vi "SAOMM-QueryHexapod.vi"(0 "PRAMMS-COMM IN":refnum<visa-resource-name>="Hp\u0000\u0002", 2 "Bool Refnum":refnum<vi>, 7 "Signature":u32=1886544237, 11 "Error IN":errorcluster, 13 "EnumMessageType":cluster{"Type":string[], "Enum":u32[]}={"Type"=["emtError", "emtAreYouThere", "emtAcknowledgment", "emtGetClientType", "emtClientType", "emtGetImageExposureTime", "emtSetImageExposureTime", "emtImageExposureTime", "emtGetOptimalExposureTime", "emtSetOptimalExposureTime", "emtOptimalExposureTime", "emtGetImageEMGain", "emtSetImageEMGain", "emtImageEMGain", "emtGetFPGACtrl", "emtSetFPGACtrl", "emtFPGACtrl", "emtGetImageWidth", "emtSetImageWidth", "emtImageWidth", "emtGetImageHeight", "emtSetImageHeight", "emtImageHeight", "emtGetImageBinning", "emtSetImageBinning", "emtImageBinning", "emtGetImageDisplayFrameRate", "emtSetImageDisplayFrameRate", "emtImageDisplayFrameRate", "emtGetROIWidth", "emtSetROIWidth", "emtROIWidth", "emtGetROIHeight", "emtSetROIHeight", "emtROIHeight", "emtGetROIXOffset", "emtSetROIXOffset", "emtROIXOffset", "emtGetROIYOffset", "emtSetROIYOffset", "emtROIYOffset", "emtStartAcquisition", "mtStopAcquisition", "emtAcquisitionStarted", "emtAcquisitionStopped", "emtGetFalconImage", "emtFalconImage"], "Enum"=[1, 2, 3, 4, 5, 1001, 1101, 1201, 1002, 1102, 1202, 1003, 1103, 1203, 1004, 1104, 1204, 1005, 1105, 1205, 1006, 1106, 1206, 1007, 1107, 1207, 1008, 1108, 1208, 1009, 1109, 1209, 1010, 1110, 1210, 1011, 1111, 1211, 1012, 1112, 1212, 1130, 1131, 1150, 1151, 1070, 1270]}) -> (4 "PRAMMS-COMM OUT":refnum<visa-resource-name>, 15 "Error OUT":errorcluster)   [LabVIEW 2019]
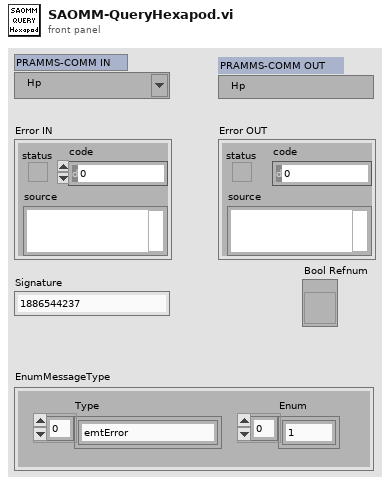
[diagram p1: front panel]
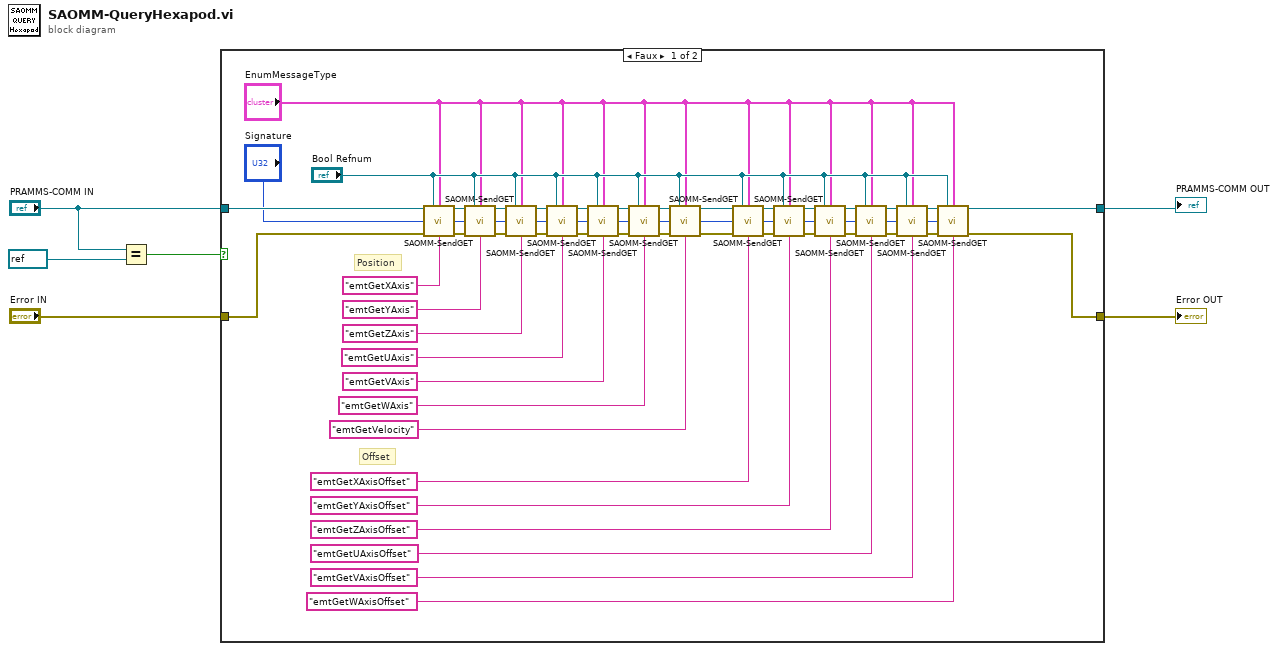
[diagram p0: block diagram]
diagram:
  n1 = Equal?(x="PRAMMS-COMM IN", y=refnum<visa-resource-name> "-1") -> (x = y?=w3:bool)
  n2 = case shown="Faux" w3 {
    tunnel: [w21 w52] -> w6
    tunnel: "PRAMMS-COMM IN" -> [w30 w52]
    tunnel: "Error IN" -> [w33 w51]
    tunnel: [w20 w51] -> w1
    frame False {
      # "Offset"
      # "Position"
      n3 = call "SAOMM-SendGET.vi"("PRAMMS-COMM IN"=w30, "Bool Refnum"="Bool Refnum", "MessageType"="EnumMessageType", "Signature"="Signature", "Error IN"=w33, "Active GET"="emtGetXAxis") -> ("PRAMMS-COMM OUT"=w31:refnum<visa-resource-name>, "Error OUT"=w32:errorcluster)  [unwired: 8 in]
      n4 = call "SAOMM-SendGET.vi"("PRAMMS-COMM IN"=w31, "Bool Refnum"="Bool Refnum", "MessageType"="EnumMessageType", "Signature"="Signature", "Error IN"=w32, "Active GET"="emtGetYAxis") -> ("PRAMMS-COMM OUT"=w45:refnum<visa-resource-name>, "Error OUT"=w41:errorcluster)  [unwired: 8 in]
      n5 = call "SAOMM-SendGET.vi"("PRAMMS-COMM IN"=w45, "Bool Refnum"="Bool Refnum", "MessageType"="EnumMessageType", "Signature"="Signature", "Error IN"=w41, "Active GET"="emtGetZAxis") -> ("PRAMMS-COMM OUT"=w44:refnum<visa-resource-name>, "Error OUT"=w40:errorcluster)  [unwired: 8 in]
      n6 = call "SAOMM-SendGET.vi"("PRAMMS-COMM IN"=w44, "Bool Refnum"="Bool Refnum", "MessageType"="EnumMessageType", "Signature"="Signature", "Error IN"=w40, "Active GET"="emtGetUAxis") -> ("PRAMMS-COMM OUT"=w43:refnum<visa-resource-name>, "Error OUT"=w39:errorcluster)  [unwired: 8 in]
      n7 = call "SAOMM-SendGET.vi"("PRAMMS-COMM IN"=w43, "Bool Refnum"="Bool Refnum", "MessageType"="EnumMessageType", "Signature"="Signature", "Error IN"=w39, "Active GET"="emtGetVAxis") -> ("PRAMMS-COMM OUT"=w42:refnum<visa-resource-name>, "Error OUT"=w38:errorcluster)  [unwired: 8 in]
      n8 = call "SAOMM-SendGET.vi"("PRAMMS-COMM IN"=w42, "Bool Refnum"="Bool Refnum", "MessageType"="EnumMessageType", "Signature"="Signature", "Error IN"=w38, "Active GET"="emtGetWAxis") -> ("PRAMMS-COMM OUT"=w36:refnum<visa-resource-name>, "Error OUT"=w35:errorcluster)  [unwired: 8 in]
      n9 = call "SAOMM-SendGET.vi"("PRAMMS-COMM IN"=w36, "Bool Refnum"="Bool Refnum", "MessageType"="EnumMessageType", "Signature"="Signature", "Error IN"=w35, "Active GET"="emtGetVelocity") -> ("PRAMMS-COMM OUT"=w23:refnum<visa-resource-name>, "Error OUT"=w22:errorcluster)  [unwired: 8 in]
      n10 = call "SAOMM-SendGET.vi"("PRAMMS-COMM IN"=w23, "Bool Refnum"="Bool Refnum", "MessageType"="EnumMessageType", "Signature"="Signature", "Error IN"=w22, "Active GET"="emtGetXAxisOffset") -> ("PRAMMS-COMM OUT"=w29:refnum<visa-resource-name>, "Error OUT"=w13:errorcluster)  [unwired: 8 in]
      n11 = call "SAOMM-SendGET.vi"("PRAMMS-COMM IN"=w29, "Bool Refnum"="Bool Refnum", "MessageType"="EnumMessageType", "Signature"="Signature", "Error IN"=w13, "Active GET"="emtGetYAxisOffset") -> ("PRAMMS-COMM OUT"=w25:refnum<visa-resource-name>, "Error OUT"=w12:errorcluster)  [unwired: 8 in]
      n12 = call "SAOMM-SendGET.vi"("PRAMMS-COMM IN"=w25, "Bool Refnum"="Bool Refnum", "MessageType"="EnumMessageType", "Signature"="Signature", "Error IN"=w12, "Active GET"="emtGetZAxisOffset") -> ("PRAMMS-COMM OUT"=w26:refnum<visa-resource-name>, "Error OUT"=w11:errorcluster)  [unwired: 8 in]
      n13 = call "SAOMM-SendGET.vi"("PRAMMS-COMM IN"=w26, "Bool Refnum"="Bool Refnum", "MessageType"="EnumMessageType", "Signature"="Signature", "Error IN"=w11, "Active GET"="emtGetUAxisOffset") -> ("PRAMMS-COMM OUT"=w27:refnum<visa-resource-name>, "Error OUT"=w10:errorcluster)  [unwired: 8 in]
      n14 = call "SAOMM-SendGET.vi"("PRAMMS-COMM IN"=w27, "Bool Refnum"="Bool Refnum", "MessageType"="EnumMessageType", "Signature"="Signature", "Error IN"=w10, "Active GET"="emtGetVAxisOffset") -> ("PRAMMS-COMM OUT"=w28:refnum<visa-resource-name>, "Error OUT"=w9:errorcluster)  [unwired: 8 in]
      n15 = call "SAOMM-SendGET.vi"("PRAMMS-COMM IN"=w28, "Bool Refnum"="Bool Refnum", "MessageType"="EnumMessageType", "Signature"="Signature", "Error IN"=w9, "Active GET"="emtGetWAxisOffset") -> ("PRAMMS-COMM OUT"=w21:refnum<visa-resource-name>, "Error OUT"=w20:errorcluster)  [unwired: 8 in]
    }
    frame True {
    }
  }
  "PRAMMS-COMM OUT" <- w6
  "Error OUT" <- w1
